vi "Attempt2.vi"() -> ()   [LabVIEW 2018]
uses:
  <vilib>/MakerHub/LINX/Public/Peripherals/Digital/Digital Write 1 Chan.vi
  <vilib>/MakerHub/LINX/Public/Peripherals/Digital/Digital Write N Chans.vi
  <vilib>/MakerHub/LINX/Private/Local IO/LinxDigitalWrite.vi
  <vilib>/MakerHub/LINX/Public/Utilities/Check Channel.vi
  <vilib>/MakerHub/LINX/Public/Utilities/Open Serial.vi
  <vilib>/MakerHub/LINX/Private/Utilties/Generate Error.vi
  <vilib>/MakerHub/LINX/LMH-LINX.lvlib
panel:
  out "Waveform":waveform(dbl)(graph)
  in  "Sampling duration (s)":dbl
  in  "Sampling freq (Hz)":dbl
  in  "Output Value":bool
  in  "Analog Channel":u8
  in  "stop":bool
  in  "Serial Port":refnum<visa-resource-name>="N/A"
  out "Error Out":errorcluster
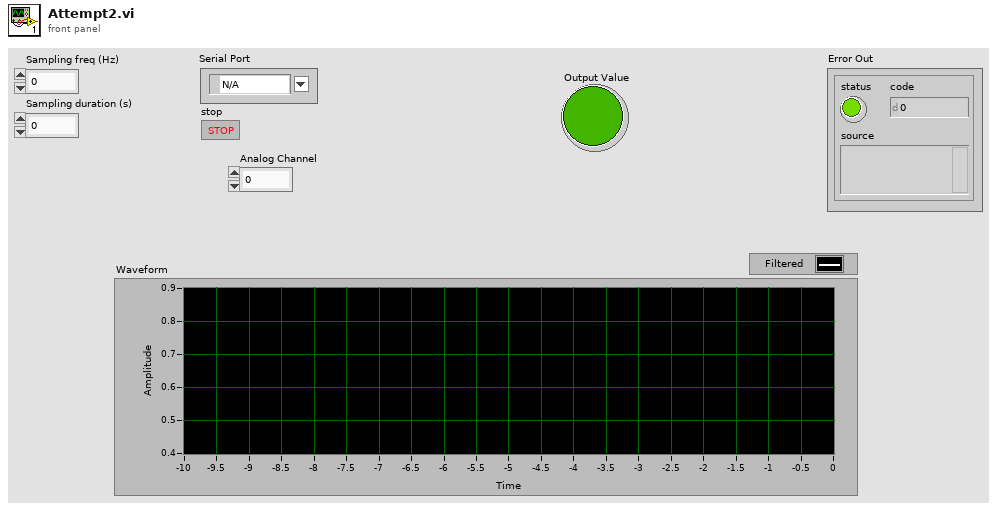
[diagram p1: front panel]
types:
  T1 = typedef "LMH-LINX.lvlib/LINX Ref.ctl" = cluster{"IO":T2, "Interface":T3, "LINX Device Config":T4}
  T2 = typedef "LMH-LINX.lvlib/Platform.ctl" = enum16{"Remote", "Local"}
  T3 = typedef "LMH-LINX.lvlib/Interface.ctl" = enum16{"Serial", "TCP"}
  T4 = typedef "LMH-LINX.lvlib/Device.lvlib/LINX Device Config.ctl" = cluster{"Interface":T3, "COM Port":refnum<visa-resource-name>, "TCP Configuration":T5, "Device Family":u8, "Device ID":u8, "Device Name":string, "TCP Ref":refnum<k5>, "Channels":T6}
  T5 = typedef "LMH-LINX.lvlib/Device.lvlib/TCP Config.ctl" = cluster{"IP Address":string, "Port":u16}
  T6 = typedef "LMH-LINX.lvlib/Channels.ctl" = cluster{"DI":u8[], "DO":u8[], "AI":u8[], "AO":u8[], "PWM":u8[], "QE":u8[], "UART":u8[], "I2C 2":u8[], "SPI":u8[], "CAN":u8[], "Servo":u8[], "AI Ref (V)":dbl, "AI Resolution (Bits)":u8, "AO Ref (V)":dbl, "AO Resolution (Bits)":u8}
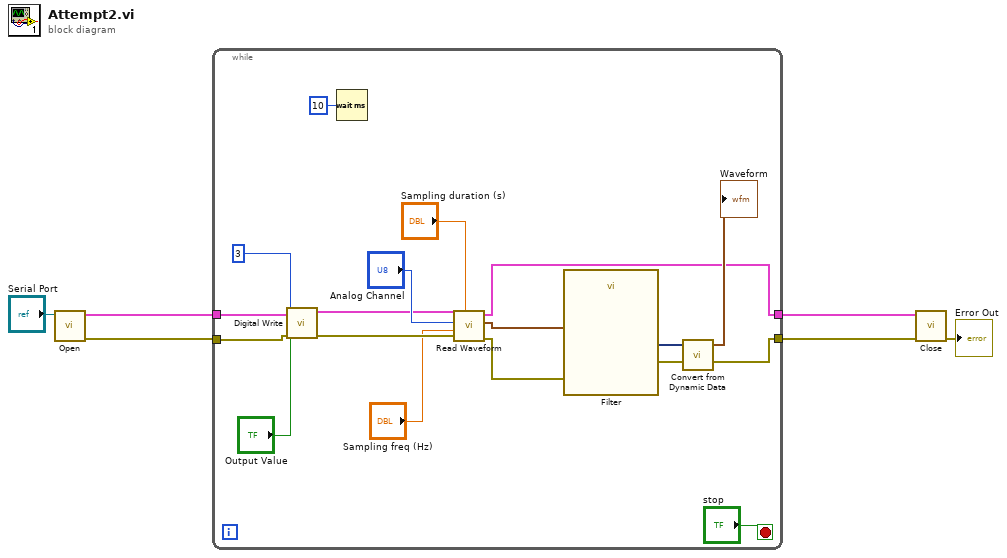
[diagram p0: block diagram]
diagram:
  n1 = call-poly <vilib>:"Open.vi"("Serial Port"="Serial Port") -> ("Error Out"=w6:errorcluster, "LINX Resource"=w5:T1)  [unwired: 8 in, 1 out]
  n2 = while {
    tunnel: w6 -> [w19]
    tunnel: w5 -> [w20]
    tunnel: [w8] -> w4
    tunnel: [w7] -> w3
    stop <- "stop" stop-if-true
    n3 = call-poly <vilib>:"Digital Write.vi"("Error In"=w19, "Output Value"="Output Value", "DO Channel"=u8 3, "LINX Resource"=w20) -> ("Error Out"=w18:errorcluster, "LINX Resource"=w17:T1)  [unwired: 6 in]
    n4 = Wait (ms)(milliseconds to wait=u32 10) -> ()  [unwired: 1 out]
    n5 = call "Read Waveform.vi"("Sampling duration (s)"="Sampling duration (s)", "error in (no error)"=w18, "Sampling freq (Hz)"="Sampling freq (Hz)", "Analog Channel"="Analog Channel", "LINX Resource in"=w17) -> ("error out"=w12:errorcluster, "Waveform out"=w11:waveform(dbl), "LINX Resource out"=w8:T1)  [unwired: 1 in, 1 out]
    n6 = call "Filter"("error in (no error)"=w12, "Signal"=w11) -> ("error out"=w7:errorcluster, "Filtered Signal"=w10:dynamicdata)  [unwired: 8 in]
    n7 = call "Convert from Dynamic Data"("Dynamic Data Type"=w10) -> ("Waveform"=→"Waveform":waveform(dbl))  [unwired: 3 in]
  }
  n8 = call <vilib>:"Close.vi"("Error In"=w3, "LINX Resource"=w4) -> ("Error Out"=→"Error Out":errorcluster)  [unwired: 9 in]
